vi "tsdiag_can_ecu_reset.vi"(8 "error in (no error)":errorcluster, 9 "mode":u8(ring)=1 items=["HardReset"=1, "keyOffOnReset"=2, "SoftReset"=3], 10 "ADiagModuleIndex":i32, 11 "path":path) -> (0 "error out":errorcluster, 1 "Success?":bool, 2 "Return Type":i32, 3 "path out":path, 5 "power down time":u8)   [LabVIEW 2014]
doc: "11服务 ECU重启。"
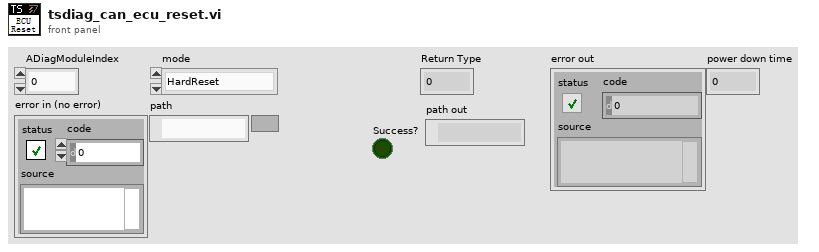
[diagram p1: front panel]
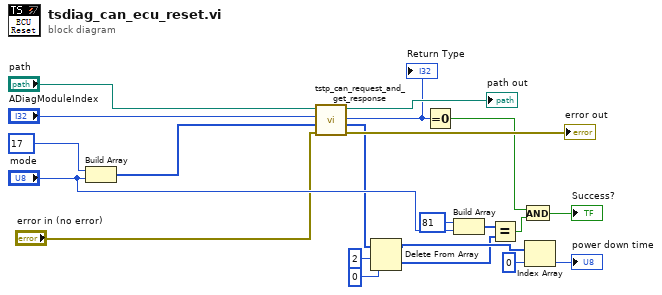
[diagram p0: block diagram]
diagram:
  n1 = Build Array(u8 17 ("element"), "mode") -> (w9:u8[])
  n2 = call "tstp_can_request_and_get_response.vi"("错误输入（无错误）"="error in (no error)", "AReqDataArray"=w9, "ADiagModuleIndex"="ADiagModuleIndex", "path"="path") -> ("错误输出"=→"error out":errorcluster, "Diagnostic response"=w4:u8[], "Return Type"=w8:i32, "path out"=→"path out":path)  [unwired: 4 in]
  "Return Type" <- w8
  n3 = Delete From Array(array=w4, length=2, index=0) -> (deleted portion=w2:u8[], array with subset deleted=w3:u8[])
  n4 = Equal To 0?(x=w8) -> (x = 0?=w7:bool)
  n5 = Build Array(u8 81 ("element"), "mode") -> (w18:u8[])
  n6 = Equal?(x=w18, y=w2) -> (x = y?=w6:bool)
  n7 = And(x=w7, y=w6) -> (x .and. y?=→"Success?":bool)
  n8 = Index Array(array=w3, index=0) -> (element=→"power down time":u8)
